vi "Tank.vi"   [LabVIEW 2012, in "Serenity_mk2.lvrbt"]
uses:
  Serenity_mk2.lvrbt
  <vilib>/NXT/Hardware/Plugins/Tetrix 180 deg Servo/Tetrix180ServoAddress.ctl
  <vilib>/NXT/Hardware/Plugins/Tetrix DC Motor/TetrixDCMotorAddress.ctl
  <vilib>/NXT/NXTIO Xnodes/NXTIONodeSubVIs/TETRIX IO Move Servos.vi
  <vilib>/NXT/NXTIO Xnodes/NXTIONodeSubVIs/TETRIX IO Move DC Motors.vi
  <vilib>/NXT/NXTIO Xnodes/NXTIONodeSubVIs/TETRIX IO Motor Status.vi
  <vilib>/NXT/NXTIO Xnodes/NXTIONodeSubVIs/TETRIX IO Check Battery.vi
  <vilib>/NXT/NXTIO Xnodes/NXTIONodeSubVIs/TETRIX IO Stop DC Motors.vi
  <vilib>/NXT/NXTIO Xnodes/AddressXNode/NXTIOAddress.xnode
  <vilib>/NXT/Subs/LVHSConnector.ctl
  <vilib>/NXT/NXTIO Xnodes/NXTIOXNode/NXTIO.xnode
  MecanumDrive/Mecanum Drive.lvrbt
  <vilib>/NXT/LegoClasses/BrickReference/BrickReference.lvclass
panel:
  # "This VI was generated based on your configuration in the Remote Control Editor. You may modify the code as needed for your robot. To test this program for an FTC match, return to the Remote Control Editor, select the \"Run Program\" tab, and choose \"Teleop\"."
types:
  T1 = typedef "Tetrix180ServoAddress.ctl" = i32
  T2 = typedef "TetrixDCMotorAddress.ctl" = i32
  T3 = cluster{"TetrixDCMotor":T2, "TetrixDCMotor 2":T2}
  T4 = typedef "LVHSConnector.ctl" = refnum<class "BrickReference.lvclass">
  T5 = typedef "FTC ControllerState.ctl" = cluster{"Left X":i8, "Left Y":i8, "Right X":i8, "Right Y":i8, "Button Encoding 9-12":u8, "Button Encoding 1-8":u8, "POV":T6}
  T6 = typedef "FTC POVState.ctl" = i8
  T7 = typedef "FTC ButtonEventType.ctl" = enum16{"Pressed", "Released"}
  T8 = cluster{"Button ID":enum16{"None", "Button 1", "Button 2", "Button 3", "Button 4", "Button 5", "Button 6", "Button 7", "Button 8", "Button 9", "Button 10", "Button 11", "Button 12", "POV Up", "POV Up Right", "POV Right", "POV Down Right", "POV Down", "POV Down Left", "POV Left", "POV Up Left"}, "Event Type":T7}[]
  T9 = typedef "FTC ButtonState.ctl" = cluster{"Button 1":bool, "Button 2":bool, "Button 3":bool, "Button 4":bool, "Button 5":bool, "Button 6":bool, "Button 7":bool, "Button 8":bool, "Button 9":bool, "Button 10":bool, "Button 11":bool, "Button 12":bool, "POV":T6}
  T10 = enum16{"None", "Button 1", "Button 2", "Button 3", "Button 4", "Button 5", "Button 6", "Button 7", "Button 8", "Button 9", "Button 10", "Button 11", "Button 12", "POV Up", "POV Up Right", "POV Right", "POV Down Right", "POV Down", "POV Down Left", "POV Left", "POV Up Left"}
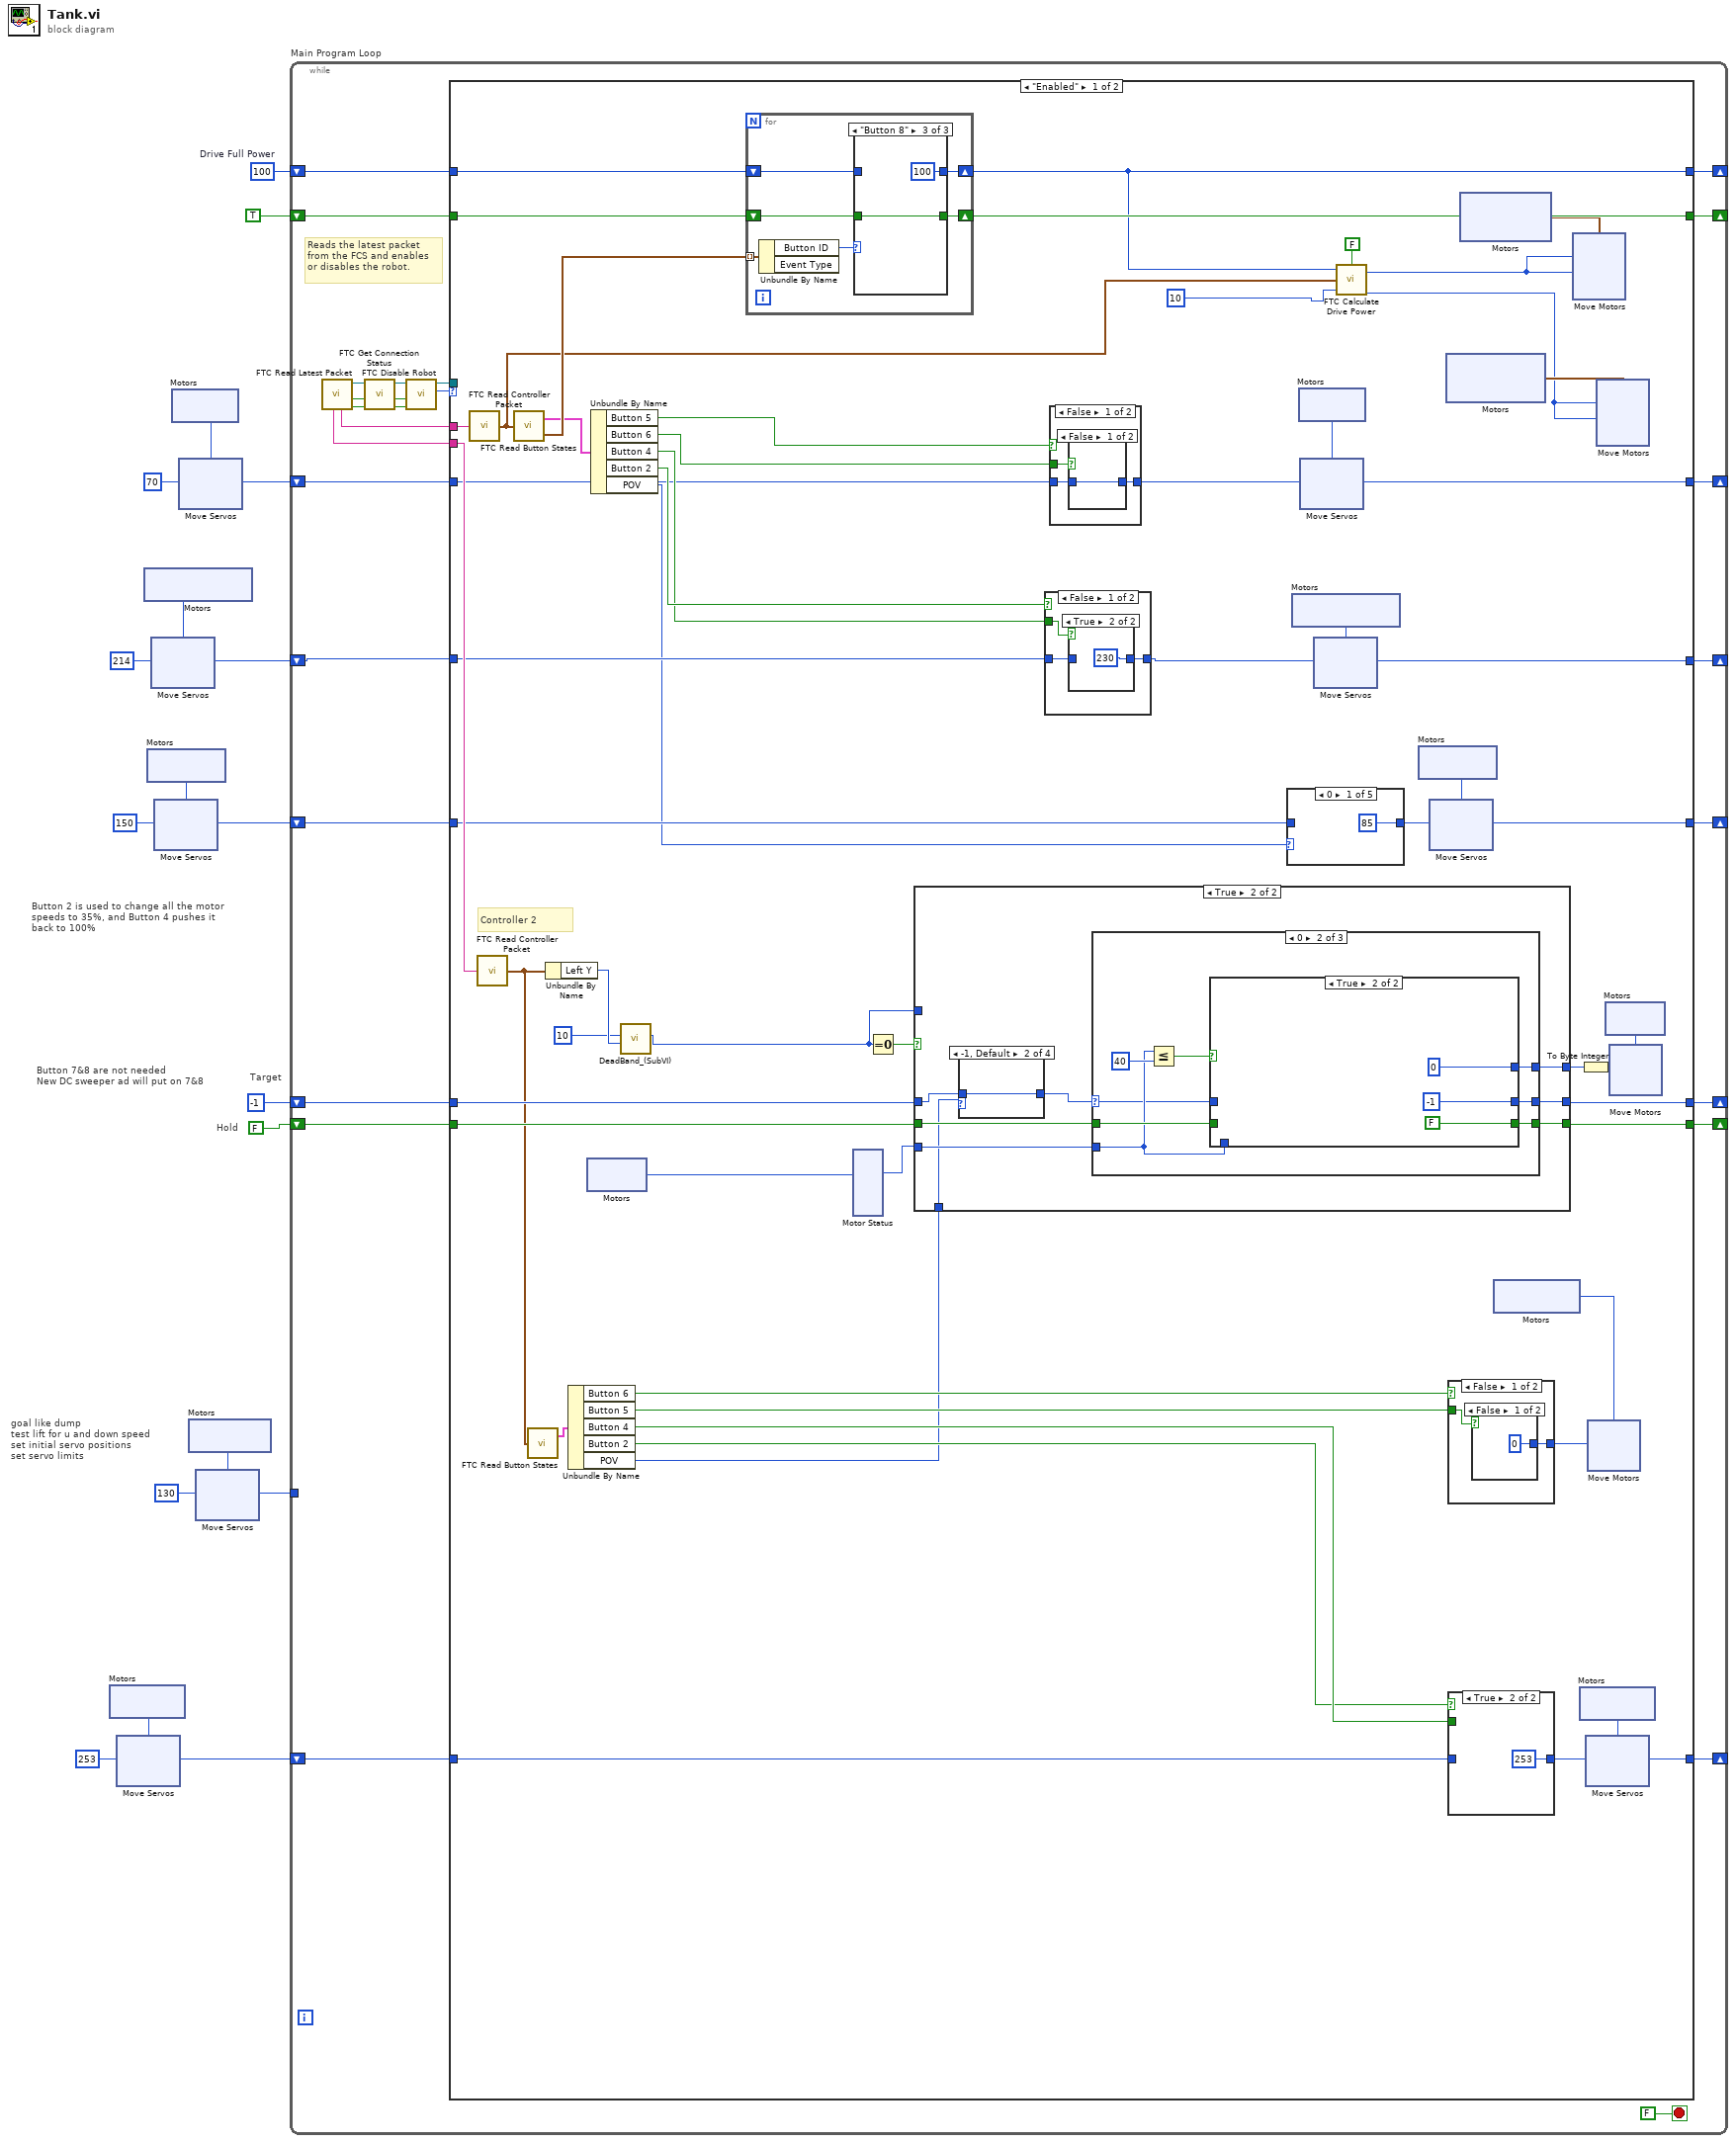
[diagram p0: block diagram]
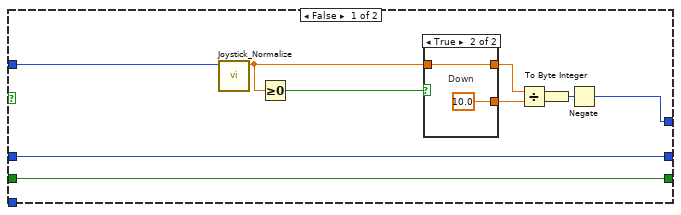
[diagram p2: hidden frame]
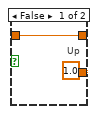
[diagram p3: hidden frame]
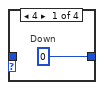
[diagram p4: hidden frame]
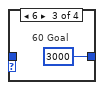
[diagram p5: hidden frame]
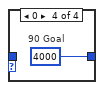
[diagram p6: hidden frame]
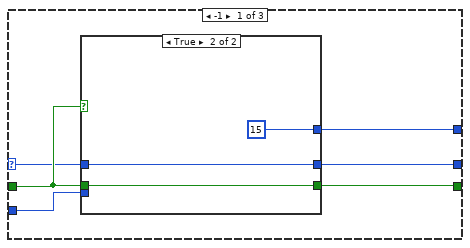
[diagram p7: hidden frame]
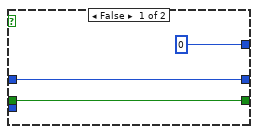
[diagram p8: hidden frame]
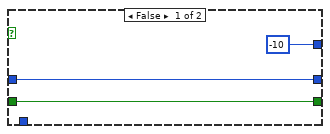
[diagram p9: hidden frame]
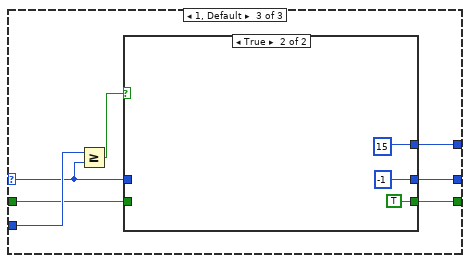
[diagram p10: hidden frame]
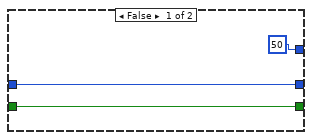
[diagram p11: hidden frame]
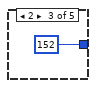
[diagram p13: hidden frame]
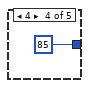
[diagram p14: hidden frame]
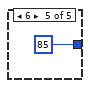
[diagram p15: hidden frame]
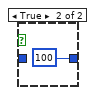
[diagram p16: hidden frame]
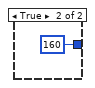
[diagram p17: hidden frame]
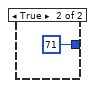
[diagram p19: hidden frame]
diagram:
  w4 = u8 150 ("Position 1")
  w5 = u8 214 ("Position 1")
  w7 = u8 70 ("Position 1")
  w11 = u8 130 ("Position 1")
  w10 = u8 253 ("Position 1")
  w14 = i8 100  # Drive Full Power
  # "Target"
  # "Hold"
  # "Button 2 is used to change all the motor \nspeeds to 35%, and Button 4 pushes it \nback to 100%"
  # "goal like dump\ntest lift for u and down speed\nset initial servo positions\nset servo limits"
  # "Button 7&8 are not needed\nNew DC sweeper ad will put on 7&8"
  n1 = xnode "Motors"() -> ("Motor"=w13:T1)
  n2 = xnode "Move Servos"("Position 1"=w10, "Motors"=w13) -> ()  [unwired: 1 in, 1 out]
  n3 = xnode "Motors"() -> ("Motor"=w6:T1)
  n4 = xnode "Motors"() -> ("Motor"=w3:T1)
  n5 = xnode "Move Servos"("Position 1"=w5, "Motors"=w6) -> ()  [unwired: 1 in, 1 out]
  n6 = xnode "Move Servos"("Position 1"=w4, "Motors"=w3) -> ()  [unwired: 1 in, 1 out]
  n7 = xnode "Motors"() -> ("Motor"=w8:T1)
  n8 = xnode "Move Servos"("Position 1"=w7, "Motors"=w8) -> ()  [unwired: 1 in, 1 out]
  n9 = xnode "Motors"() -> ("Motor"=w12:T1)
  n10 = xnode "Move Servos"("Position 1"=w11, "Motors"=w12) -> ()  [unwired: 1 in, 1 out]
  n11 = while "Main Program Loop" {
    shift-right: [w29] -> _
    shift-left: w14 -> [w30]
    tunnel: w11 -> [_]
    shift-right: [w27] -> _
    shift-left: w10 -> [w28]
    shift-right: [w25] -> _
    shift-left: TRUE -> [w26]
    shift-right: [w24] -> _
    shift-left: w7 -> [w23]
    shift-right: [w22] -> _
    shift-left: w5 -> [w21]
    shift-right: [w20] -> _
    shift-left: w4 -> [w19]
    shift-right: [w18] -> _
    shift-left: -1 -> [w17]
    shift-right: [w15] -> _
    shift-left: FALSE -> [w16]
    stop <- FALSE stop-if-true
    # "Reads the latest packet\nfrom the FCS and enables\nor disables the robot."
    n12 = call <vilib>:"FTC Read Latest Packet.vi"() -> ("Packet Received?"=w38:bool, "Stopped?"=w35:bool, "NXT"=w37:T4, "Controller 1"=w40:string, "Controller 2"=w39:string)  [unwired: 6 in, 1 out]
    n13 = call <vilib>:"FTC Get Connection Status.vi"("Packet Received?"=w38, "Stopped?"=w35, "NXT"=w37) -> ("Online?"=w32:bool, "Stopped?"=w33:bool, "NXT"=w34:T4)  [unwired: 5 in]
    n14 = call <vilib>:"FTC Disable Robot.vi"("Online?"=w32, "Stopped?"=w33, "NXT"=w34) -> ("Enabled?"=w36:enum16{"Disabled", "Enabled"}, "NXT"=w31:T4)  [unwired: 3 in]
    n15 = case "disableCase" shown="\"Enabled\"" w36 {
      tunnel: w40 -> [w95 _]
      tunnel: w39 -> [w94 _]
      tunnel: w31 -> [_ w291]
      tunnel: w30 -> [w93 w283]
      tunnel: [w71 w283] -> w29
      tunnel: w28 -> [w85 w282]
      tunnel: [w84 w282] -> w27
      tunnel: w26 -> [w81 w281]
      tunnel: [w80 w281] -> w25
      tunnel: [w60 w280] -> w24
      tunnel: w23 -> [w61 w280]
      tunnel: [w65 w279] -> w22
      tunnel: w21 -> [w64 w279]
      tunnel: [w58 w278] -> w20
      tunnel: w19 -> [w57 w278]
      tunnel: [w46 w277] -> w18
      tunnel: w17 -> [w50 w277]
      tunnel: w16 -> [w49 w276]
      tunnel: [w47 w276] -> w15
      frame "Enabled" {
        # "Controller 2"
        n16 = call <vilib>:"FTC Read Controller Packet.vi"("Packet"=w95) -> ("Controller State"=w69:T5)  [unwired: 4 in]
        n17 = call <vilib>:"FTC Read Controller Packet.vi"("Packet"=w94) -> ("Controller State"=w43:T5)  [unwired: 4 in]
        n18 = call <vilib>:"FTC Read Button States.vi"("Controller State"=w69) -> ("Button Events"=w78:T8, "Button States"=w77:T9)  [unwired: 2 in]
        n19 = call <vilib>:"FTC Read Button States.vi"("Controller State"=w43) -> ("Button States"=w87:T9)  [unwired: 2 in, 1 out]
        n20 = Unbundle By Name(w43) -> ("Left Y"=w54:i8)
        n21 = Unbundle By Name(w87) -> ("Button 6"=w92:bool, "Button 5"=w91:bool, "Button 4"=w83:bool, "Button 2"=w82:bool, "POV"=w42:T6)
        n22 = xnode "Motors"() -> ("Motor"=w45:T2)
        n23 = Unbundle By Name(w77) -> ("Button 5"=w63:bool, "Button 6"=w62:bool, "Button 4"=w66:bool, "Button 2"=w67:bool, "POV"=w56:T6)
        n24 = call "DeadBand_(SubVI).vi"("Axis In"=w54, "Deadband (10)"=i8 10) -> ("Axis out"=w51:i8)  [unwired: 9 in]
        n25 = for {
          tunnel: w78 -> [w269] mode=indexing
          shift-right: [w264] -> w71
          shift-left: w93 -> [w267]
          shift-right: [w265] -> w80
          shift-left: w81 -> [w266]
          n26 = Unbundle By Name(w269) -> ("Button ID"=w268:T10)  [unwired: 1 out]
          n27 = case shown="\"Button 8\"" w268 {
            tunnel: w267 -> [w271 _ _]
            tunnel: w266 -> [w270 w272 w274]
            tunnel: [w270 w272 w274] -> w265
            tunnel: [w271 i8 35 i8 100] -> w264
            frame "None", Default {
            }
            frame "Button 7" {
            }
            frame "Button 8" {
            }
          }
        }
        n28 = xnode "Motor Status"("Motors"=w45) -> ("Position 1"=w44:i32)  [unwired: 1 in, 2 out]
        n29 = Equal To 0?(x=w51) -> (x = 0?=w52:bool)
        n30 = case shown="True" w52 {
          tunnel: [w108 w125] -> w88
          tunnel: w51 -> [w107 _]
          tunnel: w50 -> [w106 w119]
          tunnel: w49 -> [w105 w126]
          tunnel: w44 -> [_ w124]
          tunnel: [w105 w123] -> w47
          tunnel: [w106 w122] -> w46
          tunnel: w42 -> [_ w120]
          frame False {
            n31 = call "Joystick_Normalize.vi"("Joystick In"=w107) -> ("Norm Out"=w112:sgl)  [unwired: 10 in]
            n32 = Greater Or Equal To 0?(x=w112) -> (x >= 0?=w111:bool)
            n33 = case shown="True" w111 {
              tunnel: [w116 w118] -> w109
              tunnel: w112 -> [w116 w118]
              tunnel: [sgl 1.0 sgl 10.0] -> w110
              frame False {
                # "Up"
              }
              frame True {
                # "Down"
              }
            }
            n34 = Divide(x=w109, y=w110) -> (x/y=w113:sgl)
            n35 = To Byte Integer(number=w113) -> (8bit integer=w114:i8)
            n36 = Negate(x=w114) -> (-x=w108:i8)
          }
          frame True {
            n37 = case shown="-1, Default" w120 {
              tunnel: [0 w128 3000 4000] -> w121
              tunnel: w119 -> [_ w128 _ _]
              frame 4 {
                # "Down"
              }
              frame -1, Default {
              }
              frame 6 {
                # "60 Goal"
              }
              frame 0 {
                # "90 Goal"
              }
            }
            n38 = case shown="0" w121 {
              selector: w121 -> [w132 w143 w157]
              tunnel: w126 -> [w134 w148 w160]
              tunnel: [w136 w146 w158] -> w125
              tunnel: w124 -> [w135 w145 w163]
              tunnel: [w133 w144 w159] -> w123
              tunnel: [w131 w147 w161] -> w122
              frame -1 {
                n39 = case shown="True" w134 {
                  tunnel: [0 15] -> w136
                  tunnel: w135 -> [_ _]
                  tunnel: w132 -> [w137 w141]
                  tunnel: [w137 w141] -> w131
                  tunnel: w134 -> [w138 w140]
                  tunnel: [w138 w140] -> w133
                  frame False {
                  }
                  frame True {
                  }
                }
              }
              frame 0 {
                n40 = Less Or Equal?(x=w145, y=40) -> (x <= y?=w149:bool)
                n41 = case shown="True" w149 {
                  tunnel: w148 -> [w152 _]
                  tunnel: [w152 FALSE] -> w144
                  tunnel: w143 -> [w151 _]
                  tunnel: [w151 -1] -> w147
                  tunnel: [-10 0] -> w146
                  tunnel: w145 -> [_ _]
                  frame False {
                  }
                  frame True {
                  }
                }
              }
              frame 1, Default {
                n42 = Greater Or Equal?(x=w163, y=w157) -> (x >= y?=w162:bool)
                n43 = case shown="True" w162 {
                  tunnel: [w165 -1] -> w161
                  tunnel: w157 -> [w165 _]
                  tunnel: w160 -> [w166 _]
                  tunnel: [w166 TRUE] -> w159
                  tunnel: [50 15] -> w158
                  frame False {
                  }
                  frame True {
                  }
                }
              }
            }
          }
        }
        n44 = case shown="False" w67 {
          tunnel: w66 -> [w191 _]
          tunnel: [w190 u8 71] -> w65
          tunnel: w64 -> [w189 _]
          frame False {
            n45 = case shown="True" w191 {
              tunnel: [w192 u8 230] -> w190
              tunnel: w189 -> [w192 _]
              frame False {
              }
              frame True {
              }
            }
          }
          frame True {
          }
        }
        n46 = case shown="False" w63 {
          tunnel: w62 -> [w183 _]
          tunnel: w61 -> [w184 _]
          tunnel: [w185 u8 160 ("Position 1")] -> w60
          frame False {
            n47 = case shown="False" w183 {
              tunnel: [w186 u8 100 ("lower limit")] -> w185
              tunnel: w184 -> [w186 _]
              frame False {
              }
              frame True {
              }
            }
          }
          frame True {
          }
        }
        n48 = case shown="0" w56 {
          tunnel: [u8 85 w179 u8 152 u8 85 u8 85] -> w58
          tunnel: w57 -> [_ w179 _ _ _]
          frame 0 {
          }
          frame 1, Default {
          }
          frame 2 {
          }
          frame 4 {
          }
          frame 6 {
          }
        }
        n49 = xnode "Motors"() -> ("Motor"=w68:T1)
        n50 = xnode "Motors"() -> ("Motor"=w79:T1)
        n51 = xnode "Move Servos"("Position 1"=w60, "Motors"=w79) -> ()  [unwired: 1 in, 1 out]
        n52 = xnode "Move Servos"("Position 1"=w65, "Motors"=w68) -> ()  [unwired: 1 in, 1 out]
        n53 = call-poly <vilib>:"FTC Calculate Drive Power.vi"("Reverse"=FALSE, "Deadband (10)"=i8 10, "Controller State"=w69, "Power Level (50)"=w71) -> ("Right Motor Power"=w70:i8, "Left Motor Power"=w72:i8)
        n54 = xnode "Motors"() -> ("Motor"=w59:T1)
        n55 = xnode "Move Servos"("Position 1"=w58, "Motors"=w59) -> ()  [unwired: 1 in, 1 out]
        n56 = xnode ("Motors")() -> ("Motor"=w74:cluster{"TetrixDCMotor":T2, "TetrixDCMotor":T2})
        n57 = case shown="False" w92 {
          tunnel: w91 -> [w252 _]
          tunnel: [w251 i8 -100] -> w89
          frame False {
            n58 = case shown="False" w252 {
              tunnel: [i8 0 i8 100] -> w251
              frame False {
              }
              frame True {
              }
            }
          }
          frame True {
          }
        }
        n59 = case shown="True" w82 {
          tunnel: w83 -> [w231 _]
          tunnel: [w230 u8 253] -> w84
          tunnel: w85 -> [w229 _]
          frame False {
            n60 = case shown="False" w231 {
              tunnel: [w232 u8 110] -> w230
              tunnel: w229 -> [w232 _]
              frame False {
              }
              frame True {
              }
            }
          }
          frame True {
          }
        }
        n61 = xnode ("Motors")() -> ("Motor"=w73:cluster{"TetrixDCMotor":T2, "TetrixDCMotor":T2})
        n62 = xnode "Motors"() -> ("Motor"=w90:T2)
        n63 = xnode ("Move Motors")("Power/Speed 2"=w72, "Power/Speed 1"=w72, "Motors"=w73) -> ()  [unwired: 1 in, 1 out]
        n64 = xnode "Motors"() -> ("Motor"=w86:T1)
        n65 = To Byte Integer(number=w88) -> (8bit integer=w55:i8)
        n66 = xnode "Move Servos"("Position 1"=w84, "Motors"=w86) -> ()  [unwired: 1 in, 1 out]
        n67 = xnode "Move Motors"("Power/Speed 1"=w89, "Motors"=w90) -> ()  [unwired: 1 in, 1 out]
        n68 = xnode ("Move Motors")("Power/Speed 2"=w70, "Power/Speed 1"=w70, "Motors"=w74) -> ()  [unwired: 1 in, 1 out]
        n69 = xnode "Motors"() -> ("Motor"=w48:T2)
        n70 = xnode "Move Motors"("Power/Speed 1"=w55, "Motors"=w48) -> ()  [unwired: 1 in, 1 out]
      }
      frame "Disabled" {
        # "If the robot is disabled, read the battery voltages and stop all motors."
        n71 = xnode ("Motors")() -> ("Motor"=w290:T2)
        n72 = xnode ("Check Battery")("Motors"=w290, "NXT/EV3"=w291) -> ("Voltage 1"=w289:sgl, "NXT/EV3"=w288:T4)
        n73 = xnode "Motors"() -> ("Motor"=w287:cluster{"TetrixDCMotor":T2, "TetrixDCMotor":T2})
        n74 = call <vilib>:"MCT DisplayVoltage.vi"("Motor Voltage"=w289, "NXT"=w288) -> ("NXT"=w286:T4)  [unwired: 9 in]
        n75 = xnode "Motors"() -> ("Motor"=w285:cluster{"TetrixDCMotor":T2, "TetrixDCMotor":T2})
        n76 = xnode "Stop Motors"("Motors"=w287, "NXT/EV3"=w286) -> ("NXT/EV3"=w284:T4)
        n77 = xnode "Stop Motors"("Motors"=w285, "NXT/EV3"=w284) -> ()  [unwired: 1 out]
      }
    }
  }
